vi "APS vel all.vi"(0 "Axis_ID":i32, 1 "Ve":dbl, 2 "Dec":dbl, 3 "Wait":cluster{"h_event":u32, "i32_ret":i32}, 5 "Option":i32, 7 "Vs":dbl, 9 "Vm":dbl, 11 "error in (no error)":errorcluster caption="错误输入（无错误）", 12 "Acc":dbl, 13 "SFac":dbl) -> (4 "Wait out":cluster{"h_event":u32, "i32_ret":i32}, 6 "function return":i32, 15 "error out":errorcluster caption="错误输出")   [LabVIEW 2011, in "APS168.lvlib"]
doc: "I32 FNTYPE APS_vel_all( I32 Axis_ID, I32 Option, F64 Vs, F64 Vm, F64 Ve, F64 Acc, F64 Dec, F64 SFac, ASYNCALL *Wait);"
uses:
  APS168.lvlib
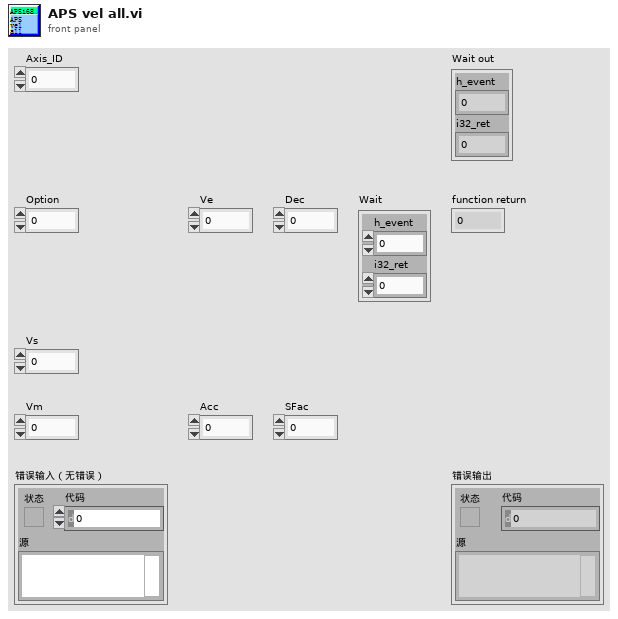
[diagram p1: front panel]
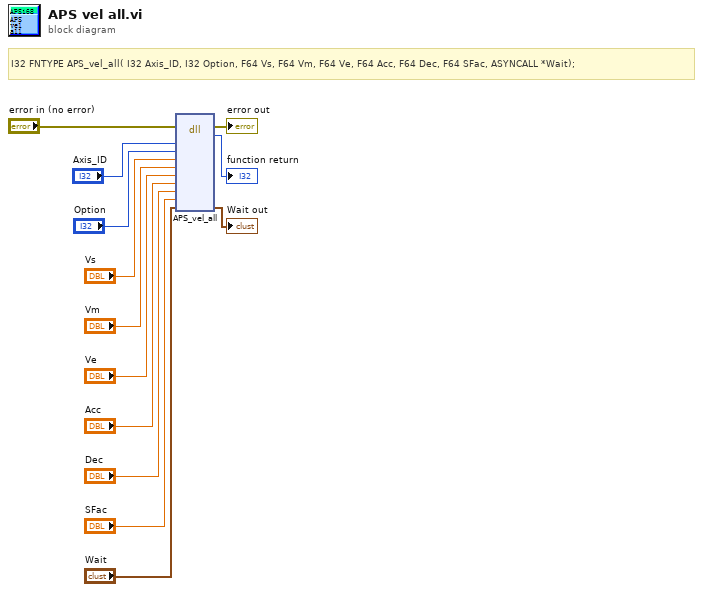
[diagram p0: block diagram]
diagram:
  # "I32 FNTYPE APS_vel_all( I32 Axis_ID, I32 Option, F64 Vs, F64 Vm, F64 Ve, F64 Acc,\tF64 Dec, F64 SFac, ASYNCALL *Wait);"
  n1 = dll-call lib="PTH1Labs E软件ADLINK 204CAPS_1_7_1_LIB line 连续运动204APS168.*" fn="APS_vel_all"(error in="error in (no error)", "Axis_ID"="Axis_ID", "Option"="Option", "Vs"="Vs", "Vm"="Vm", "Ve"="Ve", "Acc"="Acc", "Dec"="Dec", "SFac"="SFac", "Wait"="Wait") -> (error out=→"error out":errorcluster, →"function return":i32, "Wait"=→"Wait out":cluster{"h_event":u32, "i32_ret":i32})  [unwired: 10 in, 1 out]
